vi "populate.vi"(8 "error in (no error)":errorcluster, 11 "DataTypes in":refnum<class "DataTypes.lvclass">) -> (0 "error out":errorcluster, 3 "DataTypes out":refnum<class "DataTypes.lvclass">)   [LabVIEW 2018, in "DataTypes.lvclass"]
uses:
  DataTypes.lvclass
  DataTypes.lvclass/DataTypes.ctl
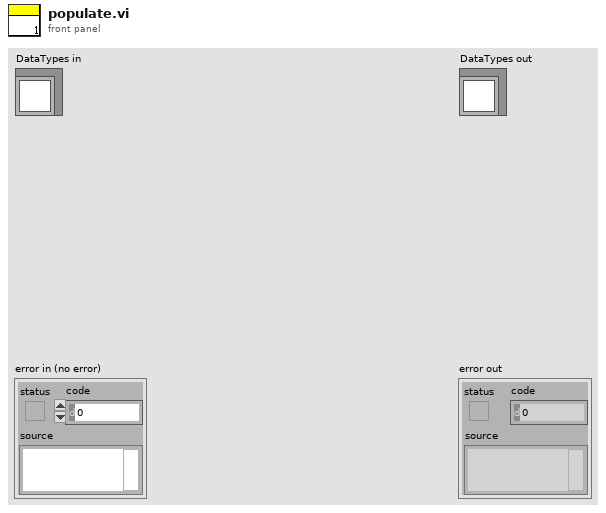
[diagram p1: front panel]
types:
  T1 = enum16{"enum-value-0", "enum-value-1", "enum-value-2"}
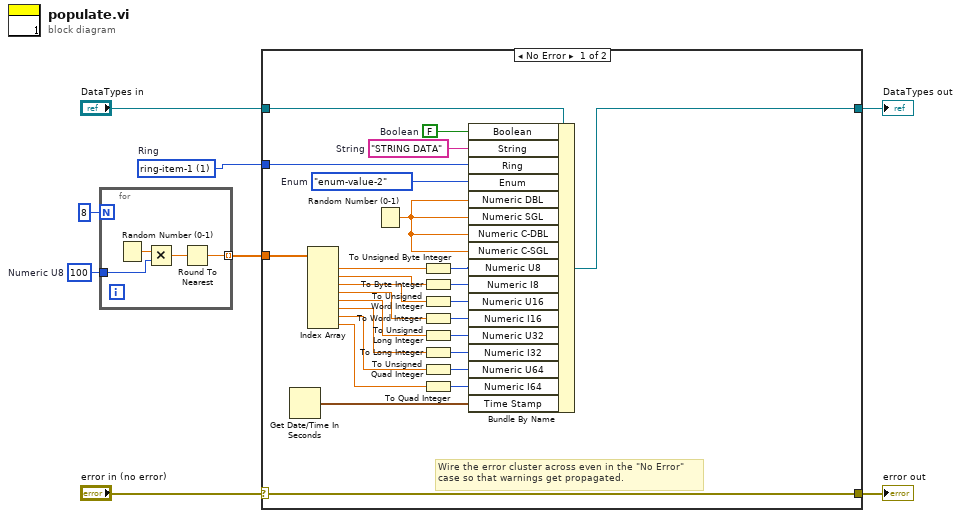
[diagram p0: block diagram]
diagram:
  w1 = u16 1 items=["ring-item-0", "ring-item-1", "ring-item-2"]  # Ring
  w3 = u8 100  # Numeric U8
  n1 = for {
    N: 8 -> [_]
    tunnel: w3 -> [w11]
    tunnel: [w9] -> w2 mode=indexing
    n2 = Random Number (0-1)() -> (number: 0 to 1=w12:dbl)
    n3 = Multiply(x=w12, y=w11) -> (x*y=w10:dbl)
    n4 = Round To Nearest(number=w10) -> (nearest integer value=w9:dbl)
  }
  n5 = case shown="No Error" "error in (no error)" {
    selector: "error in (no error)" -> [w38 w40]
    tunnel: [w38 w40] -> w7
    tunnel: [w37 w39] -> w5
    tunnel: "DataTypes in" -> [w36 w39]
    tunnel: w2 -> [w29 _]
    tunnel: w1 -> [w13 _]
    frame No Error {
      w33 = T1."enum-value-2"  # Enum
      w34 = "STRING DATA"  # String
      w35 = FALSE  # Boolean
      # "Wire the error cluster across even in the \"No Error\"\ncase so that warnings get propagated."
      n6 = Get Date/Time In Seconds() -> (seconds since 1Jan1904=w14:timestamp)
      n7 = Index Array(array=w29) -> (element #1=w28:dbl, element #2=w27:dbl, element #3=w25:dbl, element #4=w24:dbl, element #5=w22:dbl, element #6=w20:dbl, element #7=w18:dbl, element #8=w16:dbl)  [unwired: 8 in]
      n8 = Random Number (0-1)() -> (number: 0 to 1=w32:dbl)
      n9 = To Unsigned Byte Integer(number=w28) -> (unsigned 8bit integer=w30:u8)
      n10 = To Byte Integer(number=w27) -> (8bit integer=w26:i8)
      n11 = To Unsigned Word Integer(number=w25) -> (unsigned 16bit integer=w31:u16)
      n12 = To Word Integer(number=w24) -> (16bit integer=w23:i16)
      n13 = To Unsigned Long Integer(number=w22) -> (unsigned 32bit integer=w21:u32)
      n14 = To Long Integer(number=w20) -> (32bit integer=w19:i32)
      n15 = To Unsigned Quad Integer(1:w18) -> (0:w17:u64)
      n16 = To Quad Integer(1:w16) -> (0:w15:i64)
      n17 = Bundle By Name(cluster=w36, "Boolean"=w35, "String"=w34, "Ring"=w13, "Enum"=w33, "Numeric DBL"=w32, "Numeric SGL"=w32, "Numeric C-DBL"=w32, "Numeric C-SGL"=w32, "Numeric U8"=w30, "Numeric I8"=w26, "Numeric U16"=w31, "Numeric I16"=w23, "Numeric U32"=w21, "Numeric I32"=w19, "Numeric U64"=w17, "Numeric I64"=w15, "Time Stamp"=w14) -> (w37:refnum<class "DataTypes.lvclass">)
    }
    frame Error {
    }
  }
  "error out" <- w7
  "DataTypes out" <- w5
